vi "make_current.vi"(10 "VIName":string, 11 "uid":string) -> (3 "<JSON>":string)   [LabVIEW 2020]
uses:
  <vilib>/JDP Science/JSONtext/support/Format JSON Array Text.vi
  <vilib>/JDP Science/JSONtext/support/Format JSON Object.vi
  <vilib>/JDP Science/JSONtext/JSONtext.lvlib
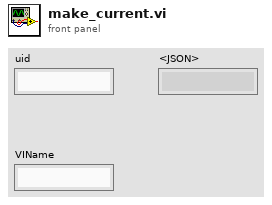
[diagram p1: front panel]
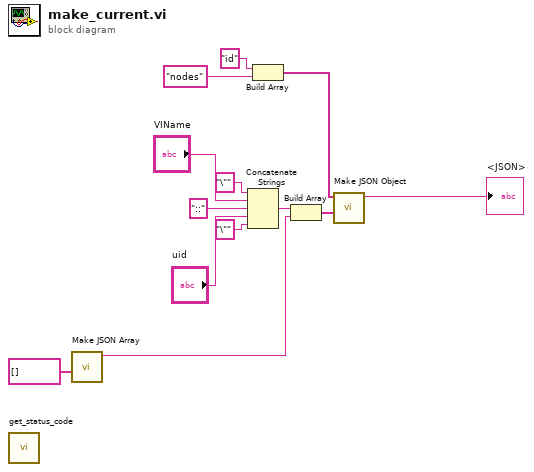
[diagram p0: block diagram]
diagram:
  n1 = call "get_status_code.vi"() -> ()  [unwired: 9 in, 2 out]
  n2 = call <vilib>:"Make JSON Array.vi"("JSON Elements"=string[] []) -> ("<JSON>"=w9:string)  [unwired: 9 in, 1 out]
  n3 = Concatenate Strings("\"" ("字符串"), "VIName", "::" ("字符串"), "uid", "\"" ("字符串")) -> (w13:string)
  n4 = Build Array("id" ("$Path or Item Name"), "nodes" ("元素")) -> (w5:string[])
  n5 = Build Array(w13, w9) -> (w6:string[])
  n6 = call <vilib>:"Make JSON Object.vi"("JSON Items"=w6, "Item Names"=w5) -> ("<JSON>"=→"<JSON>":string)  [unwired: 8 in, 1 out]
